vi "Software Update HCC List Inactive Stations.vi"(8 "error in (no error)":errorcluster, 10 "List of Stations":string[](array[string]), 11 "List of Stations 2":string[][](array[string])) -> (0 "error out":errorcluster, 3 "Array":string[][](array[string]))   [LabVIEW 2016]
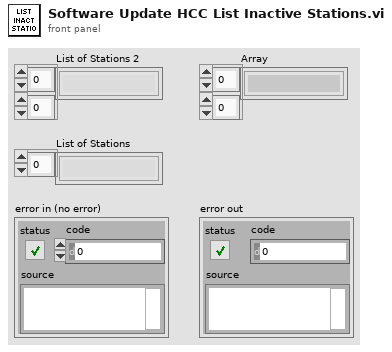
[diagram p1: front panel]
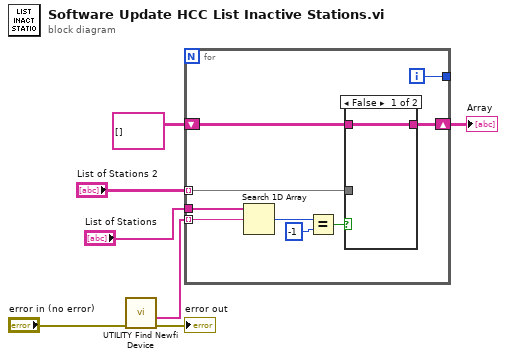
[diagram p0: block diagram]
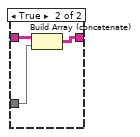
[diagram p2: hidden frame]
diagram:
  n1 = call "UTILITY Find Newfi Device.vi"("error in (no error)"="error in (no error)") -> ("error out"=→"error out":errorcluster, "Array of Newfi Devices"=w3:string[])  [unwired: 7 in, 2 out]
  n2 = for {
    tunnel: "List of Stations" -> [w16]
    tunnel: w3 -> [w15] mode=indexing
    tunnel: "List of Stations 2" -> [w9] mode=indexing
    shift-right: [w10] -> w5
    shift-left: string[][] [] -> [w11]
    tunnel: [w8] -> _
    i -> [w8]
    n3 = Search 1D Array(1D array=w16, element=w15) -> (index of element=w14:i32)  [unwired: 1 in]
    n4 = Equal?(x=w14, y=-1) -> (x = y?=w12:bool)
    n5 = case shown="False" w12 {
      tunnel: w11 -> [w17 w20]
      tunnel: [w17 w19] -> w10
      tunnel: w9 -> [_ w18]
      frame False {
      }
      frame True {
        n6 = Build Array (concatenate)(w20, w18) -> (w19:string[][])
      }
    }
  }
  "Array" <- w5
